vi "Write.vi"(8 "error in (no error)":errorcluster, 10 "String ()":string, 11 "VISA resource name":refnum<visa-resource-name>) -> (0 "error out":errorcluster, 2 "return count":i32, 3 "VISA resource name out":refnum<visa-resource-name>)   [LabVIEW 2015, in "Agilent ENA Series.lvlib"]
doc: "This VI appends linefeed to each input string and then use VISA write."
uses:
  Agilent ENA Series.lvlib
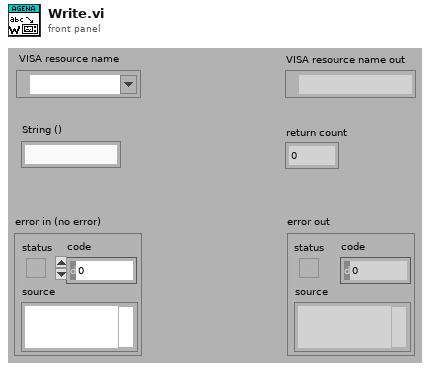
[diagram p1: front panel]
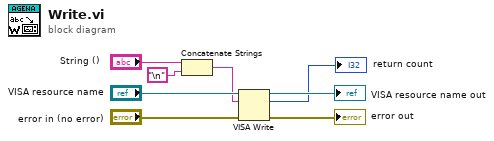
[diagram p0: block diagram]
diagram:
  n1 = Concatenate Strings("String ()", "\n") -> (w2:string)
  n2 = VISA Write(VISA resource name="VISA resource name", write buffer=w2, error in (no error)="error in (no error)") -> (VISA resource name out=→"VISA resource name out":refnum<visa-resource-name>, return count=→"return count":u32, error out=→"error out":errorcluster)
